vi "AquireTape.vi"(8 "error in (no error)":errorcluster, 11 "TapeDrive in":refnum<class "TapeDrive.lvclass">) -> (0 "error out":errorcluster, 1 "RedRatio":dbl, 2 "Settings":T1={"max velocity"={"Value"=0.0, "Min"=0.0, "Max"=0.0, "StepSize"=0.0, "Tolerance"=0.0, "ValueActual"=0.0}, "continious velocity"={"Value"=0.0, "Min"=0.0, "Max"=0.0, "StepSize"=0.0, "Tolerance"=0.0, "ValueActual"=0.0}, "shake"=enum."off", "direction"=enum."left", "RedRatio"={"Value"=0.0, "Min"=0.0, "Max"=0.0, "StepSize"=0.0, "Tolerance"=0.0, "ValueActual"=0.0}, "StepSize"={"Value"=0.0, "Min"=0.0, "Max"=0.0, "StepSize"=0.0, "Tolerance"=0.0, "ValueActual"=0.0}, "position"={"Value"=0.0, "Min"=0.0, "Max"=0.0, "StepSize"=0.0, "Tolerance"=0.0, "ValueActual"=0.0}, "velocity"={"Value"=0.0, "Min"=0.0, "Max"=0.0, "StepSize"=0.0, "Tolerance"=0.0, "ValueActual"=0.0}, "Step"=enum."off", "Mode"=enum."on demand", "timeout"={"Value"=0.0, "Min"=0.0, "Max"=0.0, "StepSize"=0.0, "Tolerance"=0.0, "ValueActual"=0.0}, "DelayStage"={"Value"=0.0, "Min"=0.0, "Max"=0.0, "StepSize"=0.0, "Tolerance"=0.0, "ValueActual"=0.0}, "TapeMotor"=enum."off", "encoder Axis"=2, "oldpos"=0.0, "ResetEncoder"=enum."off", "tape monitor"=enum."off", "ComPort"="COM1", "Stream Settings"={"My Name"="TapeDrive", "Remote IP Address"="localhost", "Remote Name"="RT"}, "Motor1Axis"=0, "Motor2Axis"=0, "OptimizeTensionAfterStep"=enum."off", "StepVelocity"={"Value"=0.0, "Min"=0.0, "Max"=0.0, "StepSize"=0.0, "Tolerance"=0.0, "ValueActual"=0.0}, "MotorDirection"=enum."left", "MinTapeMonMax"={"Value"=0.0, "Min"=0.0, "Max"=0.0, "StepSize"=0.0, "Tolerance"=0.0, "ValueActual"=0.0}, "NumberSubSteps"={"Value"=0.0, "Min"=0.0, "Max"=0.0, "StepSize"=0.0, "Tolerance"=0.0, "ValueActual"=0.0}, "SimpleMinTapeMonMaxCheck"=enum."off", "WaitBeforeScanStep"={"Value"=0.0, "Min"=0.0, "Max"=0.0, "StepSize"=0.0, "Tolerance"=0.0, "ValueActual"=0.0}, "MaxStepTries"={"Value"=100.0, "Min"=0.0, "Max"=0.0, "StepSize"=0.0, "Tolerance"=0.0, "ValueActual"=0.0}}, 3 "TapeDrive out":refnum<class "TapeDrive.lvclass">, 4 "Position (units)":dbl, 6 "velocity":dbl)   [LabVIEW 2020, in "TapeDrive.lvclass"]
uses:
  TapeDrive.lvclass
  settings_TypDef.ctl
  C:/GEECS/Developers Version/source/Device Drivers/shared/numericVariable_TypeDef.ctl
  OnOffTypeDef.ctl
  Direction_TypDef.ctl
  Mode_TypDEf.ctl
  PublicSettings.ctl
  TapeDrive.lvclass/TapeDrive.ctl
  CompressAndUpdate(Numeric).vi
  Newport ESP301.lvlib
  C:/GEECS/Developers Version/source/Device Drivers/BaseDriver/BaseDriver.lvclass
  NetworkConnection.lvclass
panel:
  out "motor2 acc gain":dbl format="%.6g"
  out "motor2 vel gain":dbl format="%.6g"
  out "motor1 acc gain":dbl format="%.6g"
  out "motor1 vel gain":dbl format="%.6g"
  out "Acceleration (units/s²) 2":dbl format="%.6g"
  out "Velocity (units/s) 2":dbl format="%.4g"
  out "Acceleration (units/s²)":dbl format="%.6g"
  out "Velocity (units/s)":dbl format="%.4g"
  in  "diags":bool
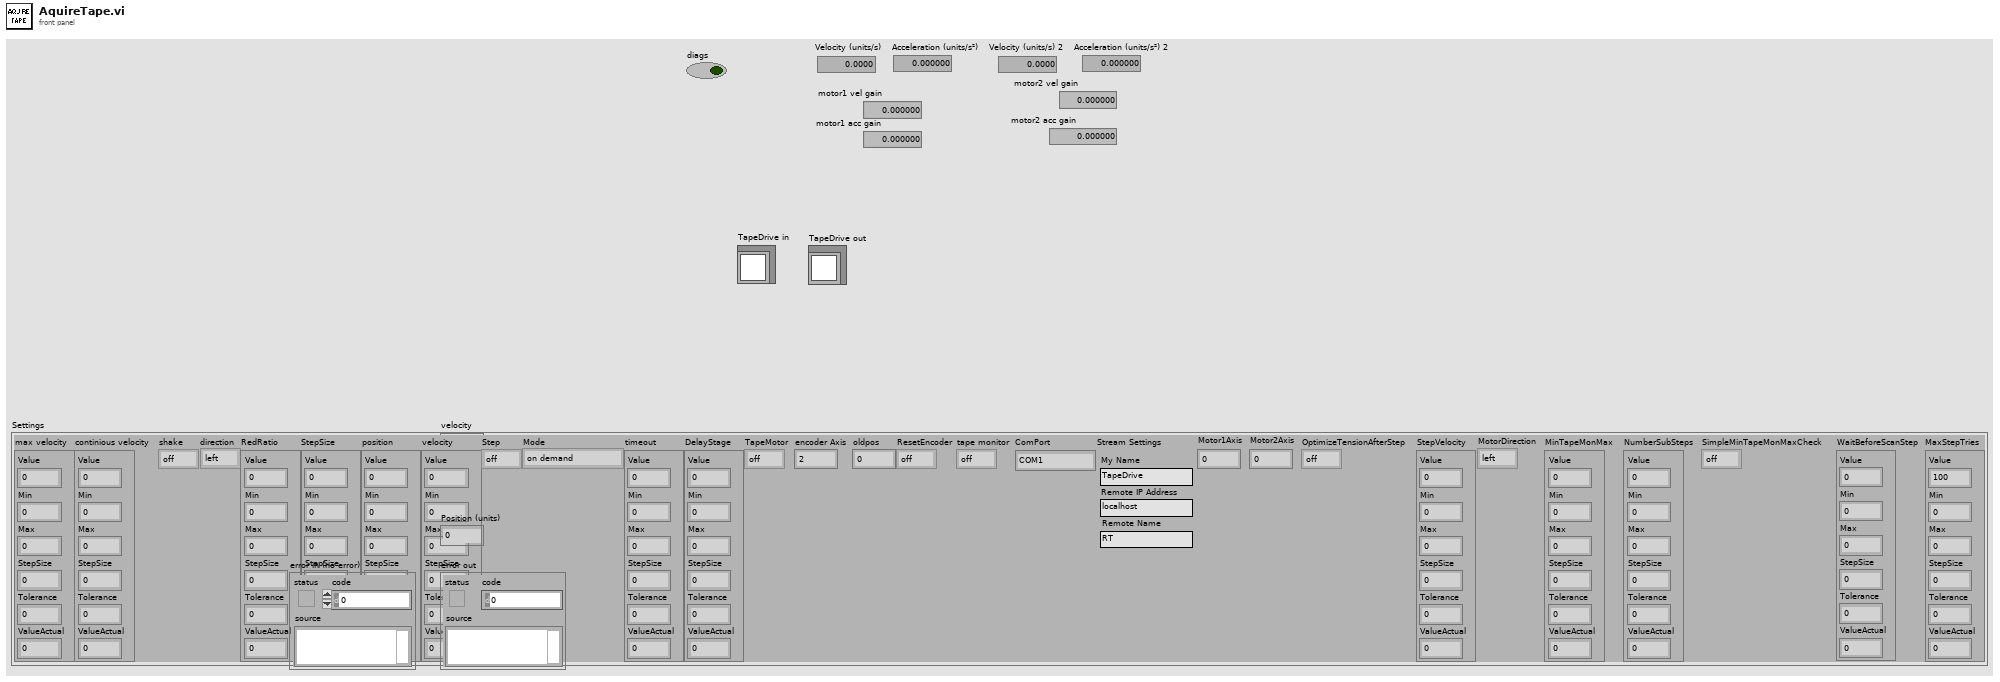
[diagram p1: front panel]
types:
  T1 = typedef "TapeDrive.lvclass/settings_TypDef.ctl" = cluster{"max velocity":T2, "continious velocity":T2, "shake":T3, "direction":T4, "RedRatio":T2, "StepSize":T2, "position":T2, "velocity":T2, "Step":T3, "Mode":T5, "timeout":T2, "DelayStage":T2, "TapeMotor":T3, "encoder Axis":i32, "oldpos":dbl, "ResetEncoder":T3, "tape monitor":T3, "ComPort":string, "Stream Settings":T6, "Motor1Axis":i32, "Motor2Axis":i32, "OptimizeTensionAfterStep":T3, "StepVelocity":T2, "MotorDirection":T4, "MinTapeMonMax":T2, "NumberSubSteps":T2, "SimpleMinTapeMonMaxCheck":T3, "WaitBeforeScanStep":T2, "MaxStepTries":T2}
  T2 = typedef "BaseDriver.lvclass/numericVariable_TypeDef.ctl" = cluster{"Value":dbl, "Min":dbl, "Max":dbl, "StepSize":dbl, "Tolerance":dbl, "ValueActual":dbl}
  T3 = typedef "OnOffTypeDef.ctl" = enum16{"off", "on"}
  T4 = typedef "Direction_TypDef.ctl" = enum16{"left", "right"}
  T5 = typedef "Mode_TypDEf.ctl" = enum16{"on demand", "continuous", "scan"}
  T6 = typedef "NetworkConnection.lvclass/PublicSettings.ctl" = cluster{"My Name":string, "Remote IP Address":string, "Remote Name":string}
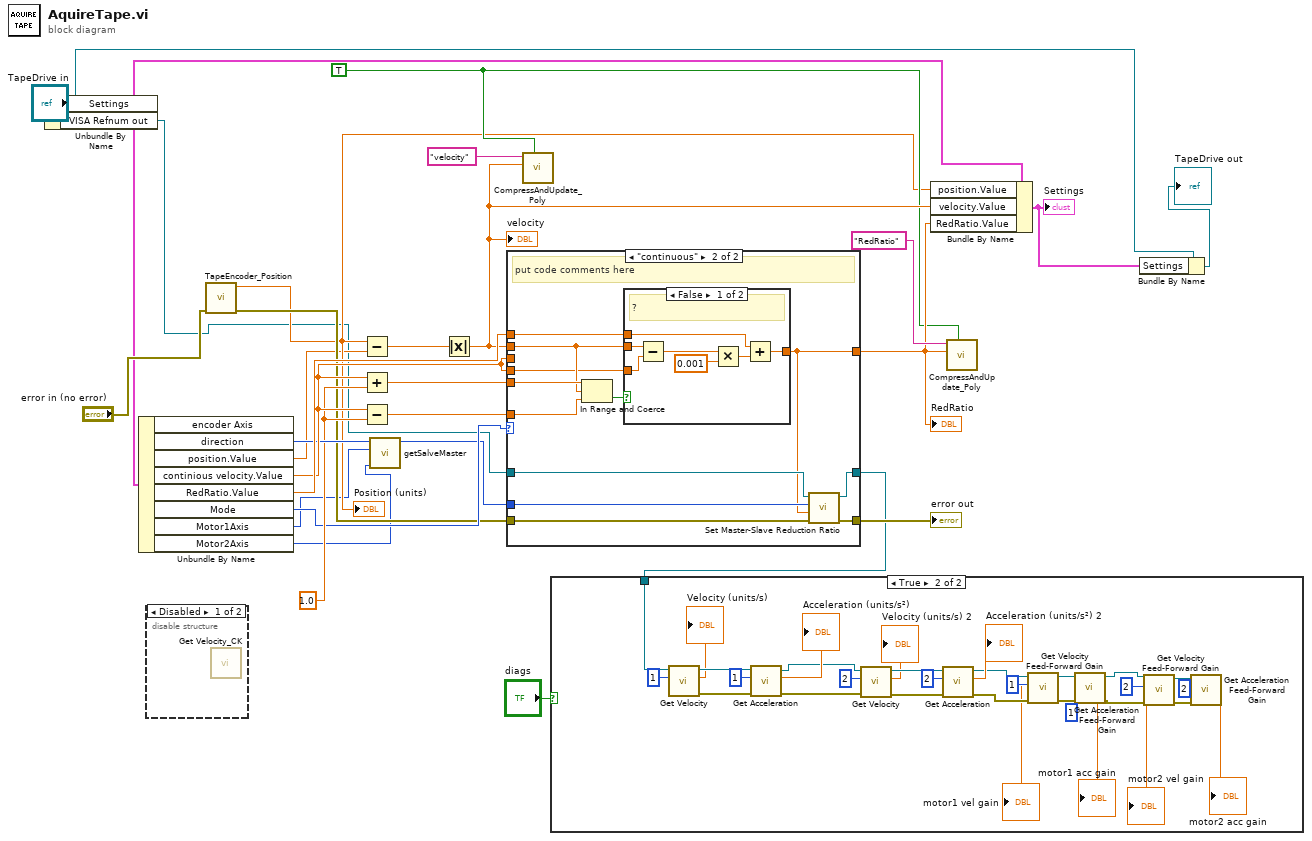
[diagram p0: block diagram]
diagram:
  w16 = TRUE ("force CVT update (false)")
  w23 = 1.0 ("y")
  n1 = Unbundle By Name("TapeDrive in") -> ("Settings"=w5:T1, "VISA Refnum out"=w1:refnum<visa-resource-name>)
  n2 = Unbundle By Name(w5) -> ("direction"=w26:T4, "position.Value"=w10:dbl, "continious velocity.Value"=w27:dbl, "RedRatio.Value"=w28:dbl, "Mode"=w15:T5, "Motor1Axis"=w9:i32, "Motor2Axis"=w8:i32)  [unwired: 1 out]
  n3 = disable-structure shown="Disabled" {
    frame Disabled {
      n4 = call "Get Velocity_CK.vi"() -> ()  [unwired: 5 in, 3 out]
    }
    frame Enabled {
    }
  }
  n5 = call "TapeEncoder_Position.vi"("error in (no error)"="error in (no error)") -> ("error IO"=w12:errorcluster, "position"=w11:dbl)  [unwired: 9 in]
  "Position (units)" <- w11
  n6 = Subtract(x=w11, y=w10) -> (x-y=w21:dbl)
  n7 = Add(x=w27, y=w23) -> (x+y=w24:dbl)
  n8 = Subtract(x=w27, y=w23) -> (x-y=w25:dbl)
  n9 = call "getSalveMaster.vi"("Motor2Axis"=w8, "Motor1Axis"=w9, "direction"=w26) -> ("Slave"=w14:i32)  [unwired: 7 in, 1 out]
  n10 = Absolute Value(x=w21) -> (abs(x)=w19:dbl)
  "velocity" <- w19
  n11 = case shown="\"continuous\"" w15 {
    tunnel: w1 -> [w31 w43]
    tunnel: [w31 w42] -> w6
    tunnel: w12 -> [w30 w41]
    tunnel: [w30 w40] -> w22
    tunnel: w14 -> [_ w39]
    tunnel: w27 -> [_ _]
    tunnel: w19 -> [_ w35]
    tunnel: w24 -> [_ w38]
    tunnel: w25 -> [_ w37]
    tunnel: w27 -> [_ w34]
    tunnel: w28 -> [w29 w33]
    tunnel: [w29 w32] -> w17
    frame "on demand", Default {
    }
    frame "continuous" {
      # "put code comments here"
      n12 = In Range and Coerce(upper limit=w38, x=w35, lower limit=w37) -> (In Range?=w36:bool)  [unwired: 1 out]
      n13 = case shown="False" w36 {
        tunnel: w35 -> [w50 _]
        tunnel: w34 -> [w49 _]
        tunnel: [w45 w51] -> w32
        tunnel: w33 -> [w44 w51]
        frame False {
          # "?"
          n14 = Subtract(x=w50, y=w49) -> (x-y=w48:dbl)
          n15 = Multiply(x=w48, y=0.001) -> (x*y=w46:dbl)
          n16 = Add(x=w44, y=w46) -> (x+y=w45:dbl)
        }
        frame True {
        }
      }
      n17 = call "Set Master-Slave Reduction Ratio.vi"("error in (no error)"=w41, "Reduction Ratio (0)"=w32, "Axis (1)"=w39, "VISA resource name"=w43) -> ("error out"=w40:errorcluster, "VISA resource name out"=w42:refnum<visa-resource-name>)  [unwired: 2 in]
    }
  }
  "RedRatio" <- w17
  "error out" <- w22
  n18 = call-poly "CompressAndUpdate_Poly.vi"("force CVT update (false)"=w16, "Numeric"=w19, "command or variable name"="velocity") -> ()  [unwired: 8 in, 1 out]
  n19 = case shown="True" "diags" {
    tunnel: w6 -> [_ w82]
    frame False {
    }
    frame True {
      n20 = call "Get Velocity.vi"("Axis (1)"=1, "VISA resource name"=w82) -> ("error out"=w70:errorcluster, "Velocity (units/s)"=→"Velocity (units/s)":dbl, "VISA resource name out"=w81:refnum<visa-resource-name>)  [unwired: 3 in]
      n21 = call "Get Acceleration.vi"("error in (no error)"=w70, "Axis (1)"=1, "VISA resource name"=w81) -> ("error out"=w69:errorcluster, "Acceleration (units/s²)"=→"Acceleration (units/s²)":dbl, "VISA resource name out"=w73:refnum<visa-resource-name>)  [unwired: 2 in]
      n22 = call "Get Velocity.vi"("error in (no error)"=w69, "Axis (1)"=2, "VISA resource name"=w73) -> ("error out"=w68:errorcluster, "Velocity (units/s)"=→"Velocity (units/s) 2":dbl, "VISA resource name out"=w74:refnum<visa-resource-name>)  [unwired: 2 in]
      n23 = call "Get Acceleration.vi"("error in (no error)"=w68, "Axis (1)"=2, "VISA resource name"=w74) -> ("error out"=w65:errorcluster, "Acceleration (units/s²)"=→"Acceleration (units/s²) 2":dbl, "VISA resource name out"=w67:refnum<visa-resource-name>)  [unwired: 2 in]
      n24 = call "Get Velocity Feed-Forward Gain.vi"("error in (no error)"=w65, "Axis (1)"=1, "VISA resource name"=w67) -> ("error out"=w58:errorcluster, "Gain"=→"motor1 vel gain":dbl, "VISA resource name out"=w61:refnum<visa-resource-name>)  [unwired: 2 in]
      n25 = call "Get Acceleration Feed-Forward Gain.vi"("error in (no error)"=w58, "Axis (1)"=1, "VISA resource name"=w61) -> ("error out"=w57:errorcluster, "Gain"=→"motor1 acc gain":dbl, "VISA resource name out"=w60:refnum<visa-resource-name>)  [unwired: 2 in]
      n26 = call "Get Velocity Feed-Forward Gain.vi"("error in (no error)"=w57, "Axis (1)"=2, "VISA resource name"=w60) -> ("error out"=w56:errorcluster, "Gain"=→"motor2 vel gain":dbl, "VISA resource name out"=w59:refnum<visa-resource-name>)  [unwired: 2 in]
      n27 = call "Get Acceleration Feed-Forward Gain.vi"("error in (no error)"=w56, "Axis (1)"=2, "VISA resource name"=w59) -> ("Gain"=→"motor2 acc gain":dbl)  [unwired: 2 in, 2 out]
    }
  }
  n28 = Bundle By Name(cluster=w5, "position.Value"=w11, "velocity.Value"=w19, "RedRatio.Value"=w17) -> (w3:T1)
  "Settings" <- w3
  n29 = call-poly "CompressAndUpdate_Poly.vi"("force CVT update (false)"=w16, "Numeric"=w17, "command or variable name"="RedRatio") -> ()  [unwired: 8 in, 1 out]
  n30 = Bundle By Name(cluster="TapeDrive in", "Settings"=w3) -> (→"TapeDrive out":refnum<class "TapeDrive.lvclass">)
